vi "加标回收率计算.vi"(11 "参数":T1) -> (2 "加标后理论浓度":dbl, 3 "参数 out":T1)   [LabVIEW 2016, in "质控单元.lvlib"]
panel:
  out "V1(mL)":dbl
  out "R":dbl
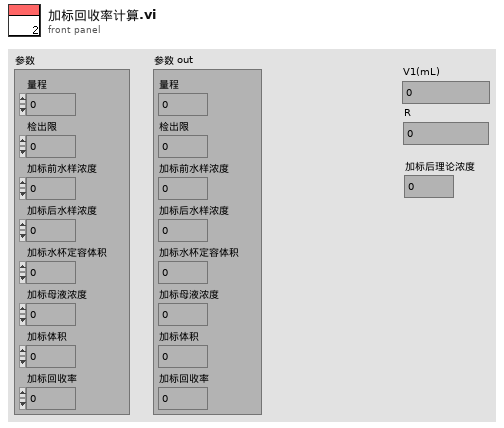
[diagram p1: front panel]
types:
  T1 = cluster{"量程":dbl, "检出限":dbl, "加标前水样浓度":dbl, "加标后水样浓度":dbl, "加标水杯定容体积":dbl, "加标母液浓度":dbl, "加标体积":dbl, "加标回收率":dbl}
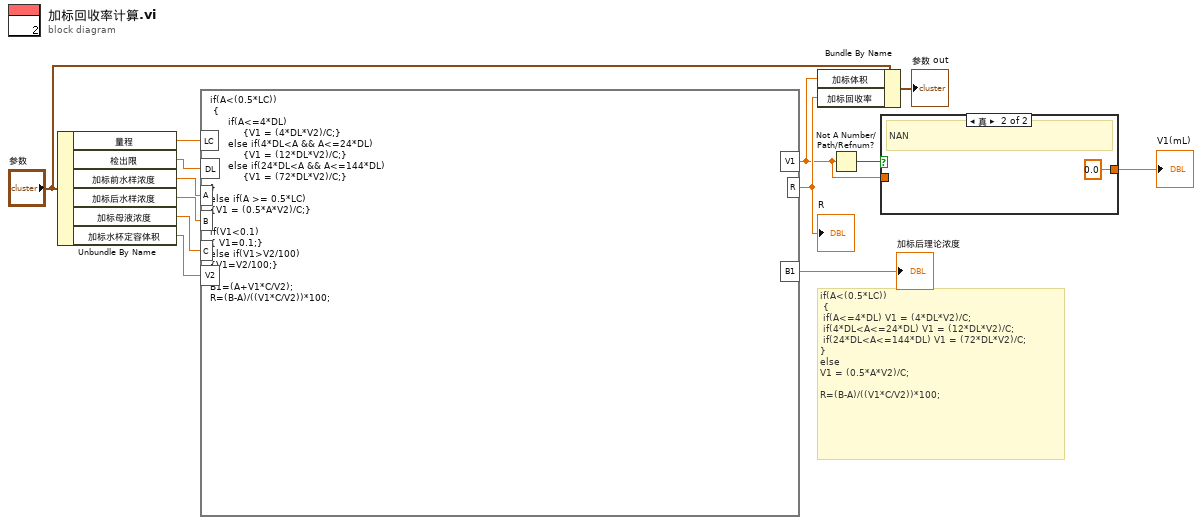
[diagram p0: block diagram]
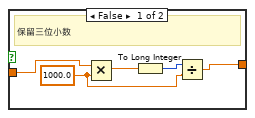
[diagram p2: hidden frame]
diagram:
  # "if(A<(0.5*LC))\n {\n if(A<=4*DL) V1 = (4*DL*V2)/C;\n if(4*DL<A<=24*DL) V1 = (12*DL*V2)/C;\n if(24*DL<A<=144*DL) V1 = (72*DL*V2)/C;\n}\nelse\nV1 = (0.5*A*V2)/C;\n\nR=(B-A)/((V1*C/V2))*100;"
  n1 = Unbundle By Name("参数") -> ("量程"=w10:dbl, "检出限"=w9:dbl, "加标前水样浓度"=w13:dbl, "加标后水样浓度"=w12:dbl, "加标母液浓度"=w11:dbl, "加标水杯定容体积"=w8:dbl)
  n2 = formula code="if(A<(0.5*LC))\n {\n      if(A<=4*DL) \n           {V1 = (4*DL*V2)/C;}\n      else if(4*DL<A && A<=24*DL) \n           {V1 = (12*DL*V2)/C;}\n      else if(24*DL<A && A<=144*DL) \n           {V1 = (72*DL*V2)/C;}\n}\nelse if(A >= 0.5*LC)\n{V1 = (0.5*A*V2)/C;}\n\nif(V1<0.1)\n{ V1=0.1;}\nelse if(V1>V2/100)\n{V1=V2/100;}\n\nB1=(A+V1*C/V2);\nR=(B-A)/((V1*C/V2))*100;"("A"=w13, "B"=w12, "C"=w11, "V2"=w8, "LC"=w10, "DL"=w9) -> ("R"=w6:dbl, "V1"=w2:dbl, "B1"=→"加标后理论浓度":dbl)
  "R" <- w6
  n3 = Bundle By Name(cluster="参数", "加标体积"=w2, "加标回收率"=w6) -> (→"参数 out":T1)
  n4 = Not A Number/Path/Refnum?(number/path/refnum=w2) -> (NaN/Path/Refnum?=w3:bool)
  n5 = case shown="真" w3 {
    tunnel: w2 -> [w18 _]
    tunnel: [w14 0.0] -> w1
    frame False {
      w15 = 1000.0 ("y")
      # "保留三位小数"
      n6 = Multiply(x=w18, y=w15) -> (x*y=w17:dbl)
      n7 = To Long Integer(number=w17) -> (32bit integer=w16:i32)
      n8 = Divide(x=w16, y=w15) -> (x/y=w14:dbl)
    }
    frame True {
      # "NAN"
    }
  }
  "V1(mL)" <- w1
